vi "Power_Test_Run.vi"() -> ()   [LabVIEW 2021]
uses:
  <vilib>/DAQmx/read.llb/DAQmx Read (Analog 1D Wfm NChan NSamp).vi
  <vilib>/DAQmx/miscellaneous.llb/DAQmx Fill In Error Info.vi
  <vilib>/measure/madcrms.llb/Averaged DC-RMS for N Chan.vi
  <vilib>/measure/madcrms.llb/Basic Averaged DC-RMS for N Chan.vi
  <vilib>/measure/NI_MAPro.lvlib
panel:
  out "XY Graph":cluster{dbl[], dbl[]}(graph)
  out "Raw Readings 2":waveform(dbl)[](graph)
  out "Frequency":cluster{dbl[], dbl[]}(graph)
  out "XY Graph 2":cluster{dbl[], dbl[]}(graph)
  out "Array 2":dbl[](array[numeric])
  out "Avg VRMS":dbl[](graph)
  out "VRMS Sine":dbl[][](graph)
  out "data":waveform(dbl)[][](array[waveform])
  in  "?":bool
  out "DC values":dbl[](array[numeric]) format="%.2p"
  out "RMS values":dbl[](array[numeric]) format="%.2p"
  out "Raw Readings":waveform(dbl)[](graph)
  in  "millisecond multiple":u32
  out "DC value waveforms":waveform(dbl)[](array[waveform])
  out "RMS value waveforms":waveform(dbl)[](array[waveform])
  in  "error in":errorcluster
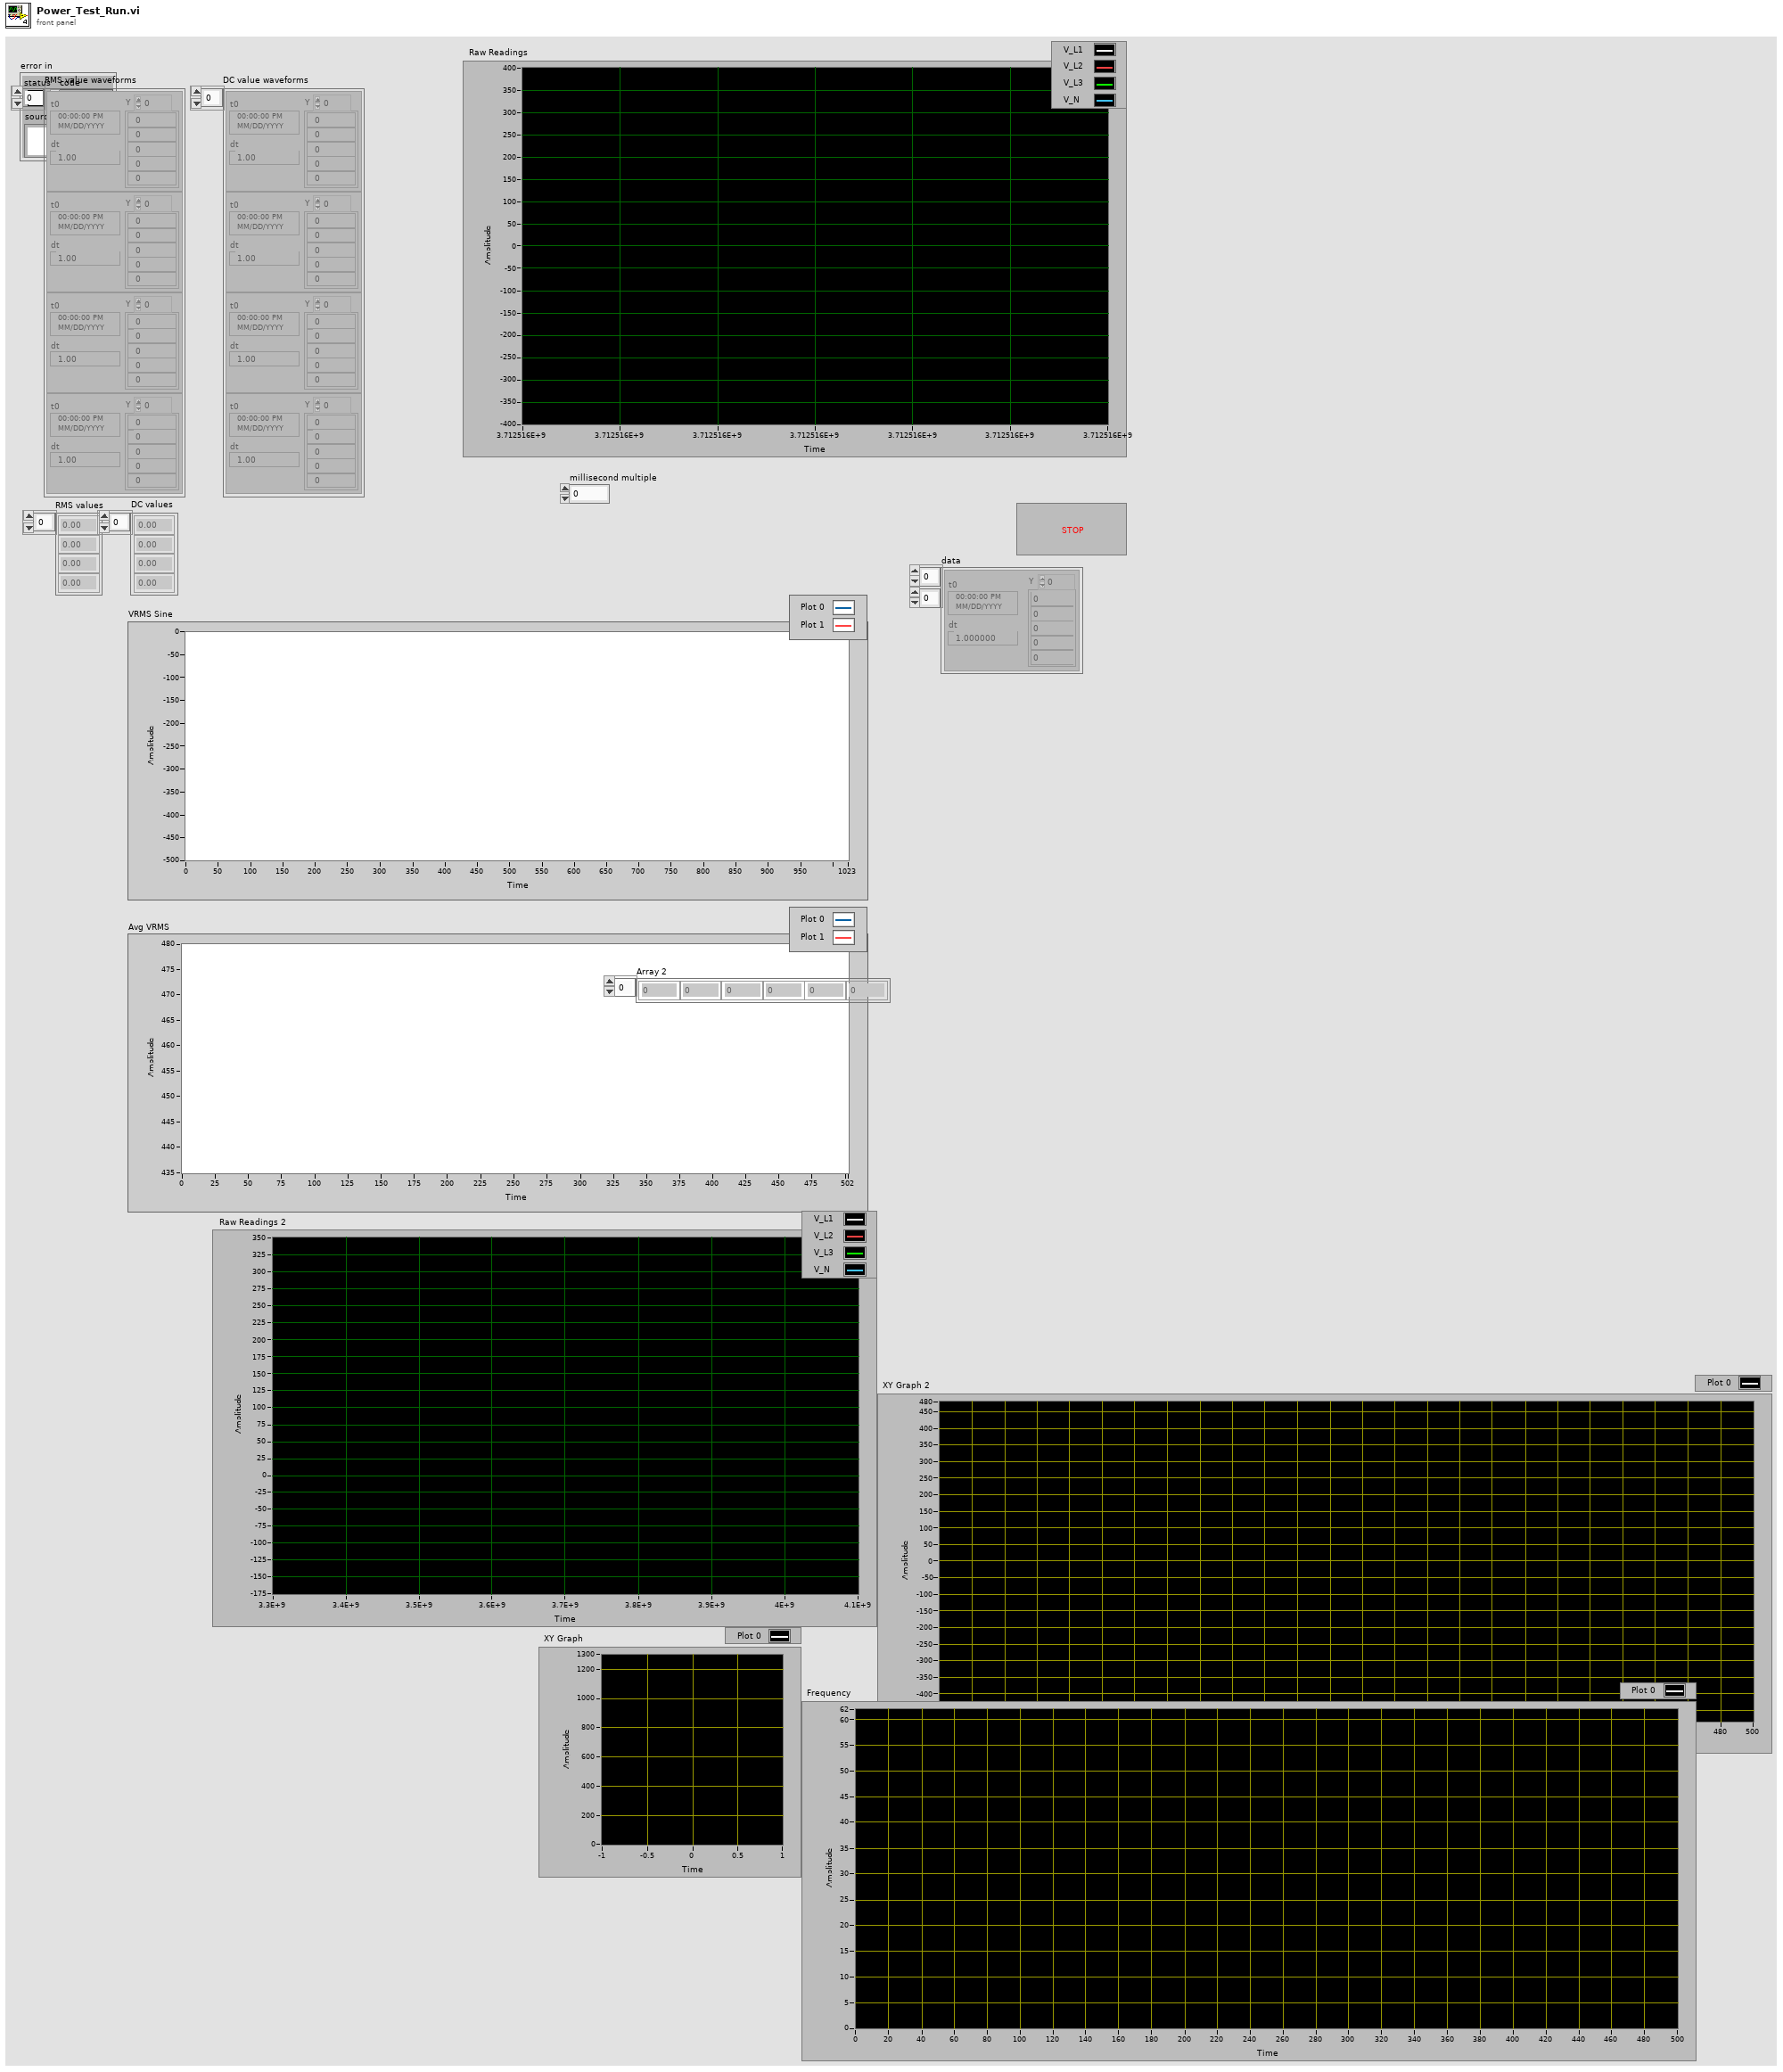
[diagram p1: front panel]
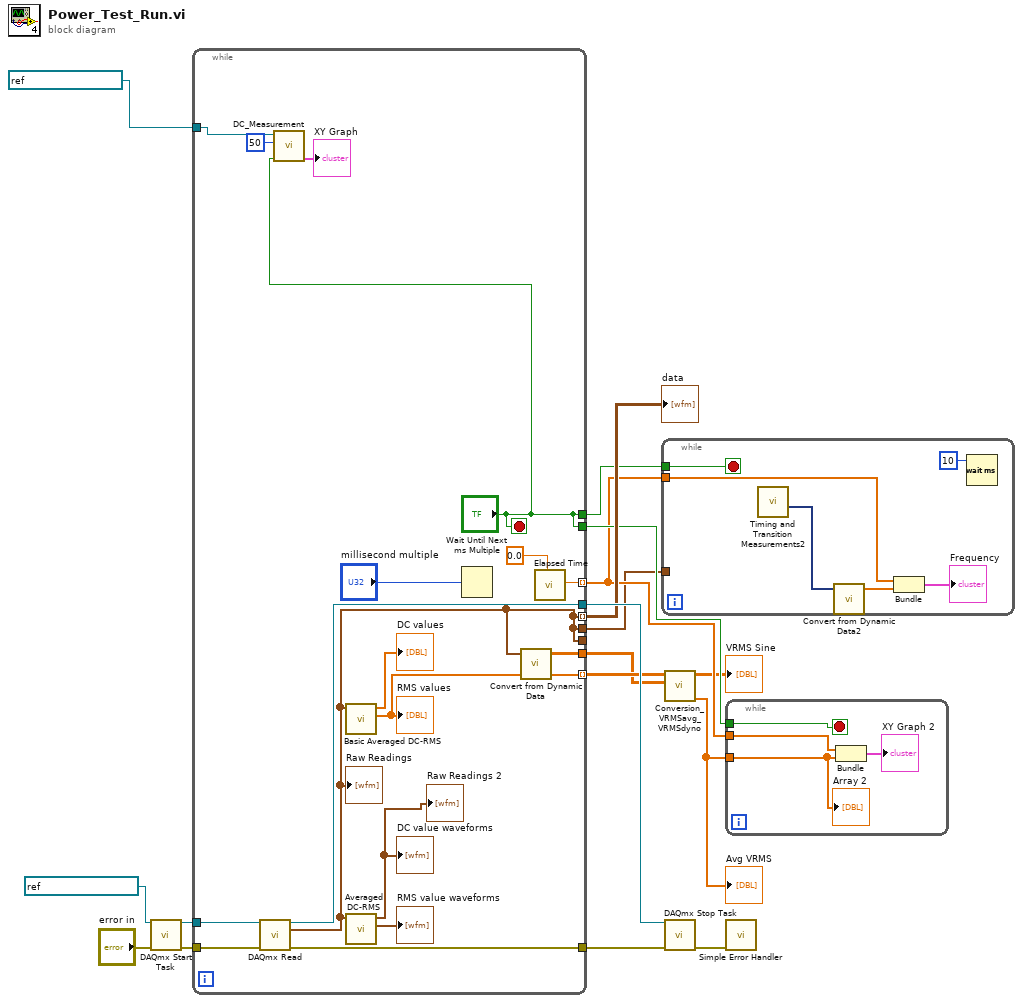
[diagram p0: block diagram]
diagram:
  n1 = call <vilib>:"DAQmx Start Task.vi"("task/channels in"=refnum<k21> "PTS_Cab1k_9244", "error in"="error in") -> ("task out"=w16:refnum<k21>, "error out"=w14:errorcluster)  [unwired: 12 in]
  n2 = while {
    tunnel: w14 -> [w33]
    tunnel: [w32] -> w13
    tunnel: w16 -> [w24]
    tunnel: [w34] -> w15
    tunnel: [w29] -> w9 mode=indexing
    tunnel: [w23] -> w10 mode=indexing
    tunnel: [w27] -> w8
    tunnel: [w23] -> _
    tunnel: [w25] -> w5 mode=indexing
    tunnel: ["?"] -> w7
    tunnel: ["?"] -> w4
    tunnel: [w23] -> w2
    tunnel: refnum<k21> "PTS_Cab1k_9205" ("task/channels in") -> [w19]
    stop <- "?" stop-if-true
    n3 = call-poly <vilib>:"DAQmx Read.vi"("task/channels in"=w24, "error in"=w33) -> ("task out"=w34:refnum<k21>, "data"=w23:waveform(dbl)[], "error out"=w32:errorcluster)  [unwired: 11 in]
    "Raw Readings" <- w23
    n4 = call "DC_Measurement.vi"("stop"="?", "millisecond multiple"=u32 50, "task/channels in"=w19) -> ("XY Graph"=→"XY Graph":cluster{dbl[], dbl[]})  [unwired: 8 in]
    n5 = call-poly <vilib>:"Basic Averaged DC-RMS.vi"("signals in"=w23) -> ("RMS values"=w29:dbl[], "DC values"=→"DC values":dbl[])  [unwired: 7 in, 2 out]
    "RMS values" <- w29
    n6 = call-poly <vilib>:"Averaged DC-RMS.vi"("signals in"=w23) -> ("RMS value waveforms"=→"RMS value waveforms":waveform(dbl)[], "DC value waveforms"=→"DC value waveforms" →"Raw Readings 2":waveform(dbl)[])  [unwired: 6 in, 3 out]
    n7 = Wait Until Next ms Multiple(millisecond multiple="millisecond multiple") -> ()  [unwired: 1 out]
    n8 = call "Convert from Dynamic Data"("Dynamic Data Type"=w23) -> ("Array"=w27:dbl[][])  [unwired: 3 in]
    n9 = call "Elapsed Time"("Set Start Time (s)"=0.0) -> ("Elapsed Time (s)"=w25:dbl)  [unwired: 11 in, 7 out]
  }
  "data" <- w10
  n10 = while {
    tunnel: w4 -> [w40]
    tunnel: w5 -> [w38]
    tunnel: w2 -> [_]
    stop <- w40 stop-if-true
    n11 = call "Timing and Transition Measurements2"() -> ("Frequency"=w36:dynamicdata)  [unwired: 10 in, 1 out]
    n12 = call "Convert from Dynamic Data2"("Dynamic Data Type"=w36) -> ("Array"=w37:dbl[])  [unwired: 3 in]
    n13 = Bundle(w38, "Array"=w37) -> (→"Frequency":cluster{dbl[], "Array":dbl[]})  [unwired: 1 in]
    n14 = Wait (ms)(milliseconds to wait=u32 10) -> ()  [unwired: 1 out]
  }
  n15 = call "Conversion_VRMSavg_VRMSdyno.vi"("Dynamic Data"=w8, "VRMS"=w9) -> ("VRMS Avg"=w6:dbl[], "VRMS Sine"=→"VRMS Sine":dbl[][])  [unwired: 8 in]
  "Avg VRMS" <- w6
  n16 = call <vilib>:"DAQmx Stop Task.vi"("task/channels in"=w15, "error in"=w13) -> ("error out"=w12:errorcluster)  [unwired: 12 in, 1 out]
  n17 = while {
    tunnel: w7 -> [w44]
    tunnel: w5 -> [w42]
    tunnel: w6 -> [w41]
    stop <- w44 stop-if-true
    n18 = Bundle(w42, "VRMS Avg"=w41) -> (→"XY Graph 2":cluster{dbl[], "VRMS Avg":dbl[]})  [unwired: 1 in]
    "Array 2" <- w41
  }
  n19 = call <vilib>:"Simple Error Handler.vi"("error in (no error)"=w12) -> ()  [unwired: 4 in, 5 out]
